vi "BasicTestWithIFw.vi"() -> ()   [LabVIEW 2015]
uses:
  SVPWM/SwitchPositions.ctl
  <vilib>/Platform/TimedLoop/XDataNode/timing_clust.ctl
  <vilib>/Platform/TimedLoop/XDataNode/nitl_modes.ctl
  <vilib>/Platform/TimedLoop/XDataNode/wakeup.ctl
  <vilib>/rvi/FXPMathLib/FxpSinAndCos/subVIs/nifxpmath_SinAndCos_SimConfig.ctl
  <vilib>/rvi/Emulation/niFpgaGetClockAttributes.vi
  <vilib>/rvi/Emulation/niFpgaSctlEmulationGetInTimedLoop.vi
  <vilib>/rvi/Emulation/niFpgaEmulationReportErrorSimple.vi
  <vilib>/rvi/FXPMathLib/FxpSinAndCos/simVIs/DllFxpSinAndCosTemp_sub.vi
  <vilib>/rvi/Emulation/niFpgaProcessEmulError.vi
  <vilib>/rvi/Emulation/niFpgaCriticalErrorInLSC.vi
  <vilib>/rvi/DataTransferAndStorage/Container/Common/niFpgaContainerExecOnDevCompGetState.vi
  <vilib>/rvi/Emulation/niFpgaEmulationIsFPGAContextNoSignature.vi
  <vilib>/rvi/DataTransferAndStorage/Container/Common/niFpgaContainerGetUniqueNameForEmu.vi
  <vilib>/rvi/Memory/Memory_Emulation/niFpgaMemoryEmulationCacheClearOnFirstRun.vi
  <vilib>/rvi/Memory/Memory_Emulation/nirvimemoryEmulationManagerCache_MakeExclusive.vi
  <vilib>/rvi/Memory/Memory_Emulation/niFpgaMemoryEmulationValidateCache.vi
  <vilib>/rvi/Memory/Memory_Emulation/nirvimemoryEmulationManagerCache_InsertValue.vi
  <vilib>/Utility/error.llb/Clear Errors.vi
  <vilib>/rvi/Memory/Memory_Emulation/nirvimemoryEmulationManagerCache_ReleaseExclusive.vi
  <vilib>/rvi/Memory/Memory_Emulation/nirvimemoryEmulationManagerCache_GetValue.vi
  <vilib>/rvi/Memory/Memory_Emulation/nirvimemoryEmulationManagerCache_SetValue.vi
  <vilib>/rvi/eio/common/nirviEmuTemplateMethod_errors.vi
  <vilib>/rvi/FXPMathLib/FxpSinAndCos/XNode/nifxpmath_SinAndCos.xnode
  <vilib>/Platform/TimedLoop/XDataNode/XDataNode.xnode
  <vilib>/rvi/DataTransferAndStorage/Container/XNode/niFpgaContainer.xnode
  <vilib>/rvi/DataTransferAndStorage/Register/Emulation/niFpgaRegisterEmulationRefIn.vi
  <vilib>/eio/EIONode/EIONode.xnode
  <vilib>/Platform/TimedLoop/XDataNode/XDNodeRunTimeDep.lvlib
  SVPWM/SVPWM.lvlib
  SVPWM/AddressSpace.lvclass
  <instrlib>/_niInstr/Instruction Framework/v1/FPGA/Top Level Bus/Register Configuration/Register Configuration.lvclass
  <instrlib>/_niInstr/FIFO Register Bus/v1/FPGA/niInstr FIFO Register Bus v1 FPGA.lvclass
panel:
  out "Period":u32
  out "Deadtime":u8
  in  "fifo reg bus ctrl 0":u32
  out "fifo reg bus status 0":u32
  out "fifo reg bus data 0":u64
  out "SwitchPositions":T1
  out "Sector":u8
  in  "enable":bool
  in  "engauge":bool
  in  "freq":sgl
  in  "modulation":fxp<+/-,16,2>=1.0
  out "As":sgl
  out "Bs":sgl
  out "Cs":sgl
  out "alpha":sgl
  out "beta":sgl
  in  "Count(Ticks)":u32=400
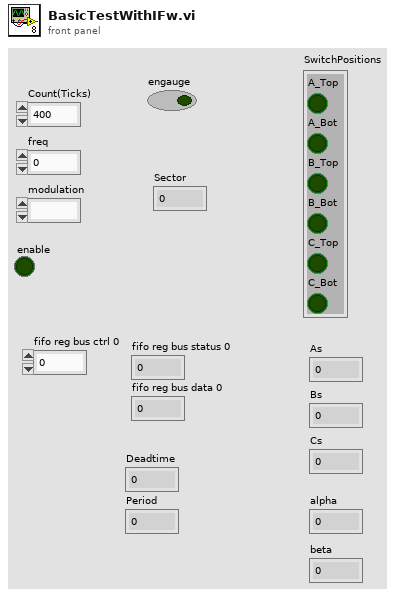
[diagram p1: front panel]
types:
  T1 = typedef "SVPWM.lvlib/SwitchPositions.ctl" = cluster{"A_Top":bool, "A_Bot":bool, "B_Top":bool, "B_Bot":bool, "C_Top":bool, "C_Bot":bool}
  T2 = typedef "XDNodeRunTimeDep.lvlib/timing_clust.ctl" = cluster{"Expected End [f-1]":u64, "Actual End [f-1]":u64, "Finished Late? [f-1]":bool, "Expected End [i-1]":u64, "Actual End [i-1]":u64, "Finished Late? [i-1]":bool, "Expected Start [i]":u64, "Actual Start [i]":u64, "Expected Start [f]":u64, "Actual Start [f]":u64, "Source Name":string, "Structure Name":string, "Period":i64, "Deadline":i64, "Offset":i64, "Start":i64, "Priority":i32, "Timeout":i32, "Mode":T3, "Wakeup Reason":T4, "Error":errorcluster, "Source Type":string, "Secondary Source Type":string, "Global End Time":u64, "Global Start Time":u64, "Frame Duration":u64, "Iteration Duration":u64, "Assigned CPU":i32, "I/O Scan Engine Mode":u32}
  T3 = typedef "XDNodeRunTimeDep.lvlib/nitl_modes.ctl" = enum32{"No Change", "Process missed periods, maintain original phase", "Discard missed periods, maintain original phase", "Process missed periods, ignore original phase", "Discard missed periods, ignore original phase"}
  T4 = typedef "XDNodeRunTimeDep.lvlib/wakeup.ctl" = enum32{"Normal", "Aborted", "Asynchronous wakeup", "Timing source error", "Timed loop error", "Timeout"}
  T5 = typedef "SVPWM.lvlib/Parameters.ctl" = cluster{"Deadtime":refnum<k21>, "Period":refnum<k21>}
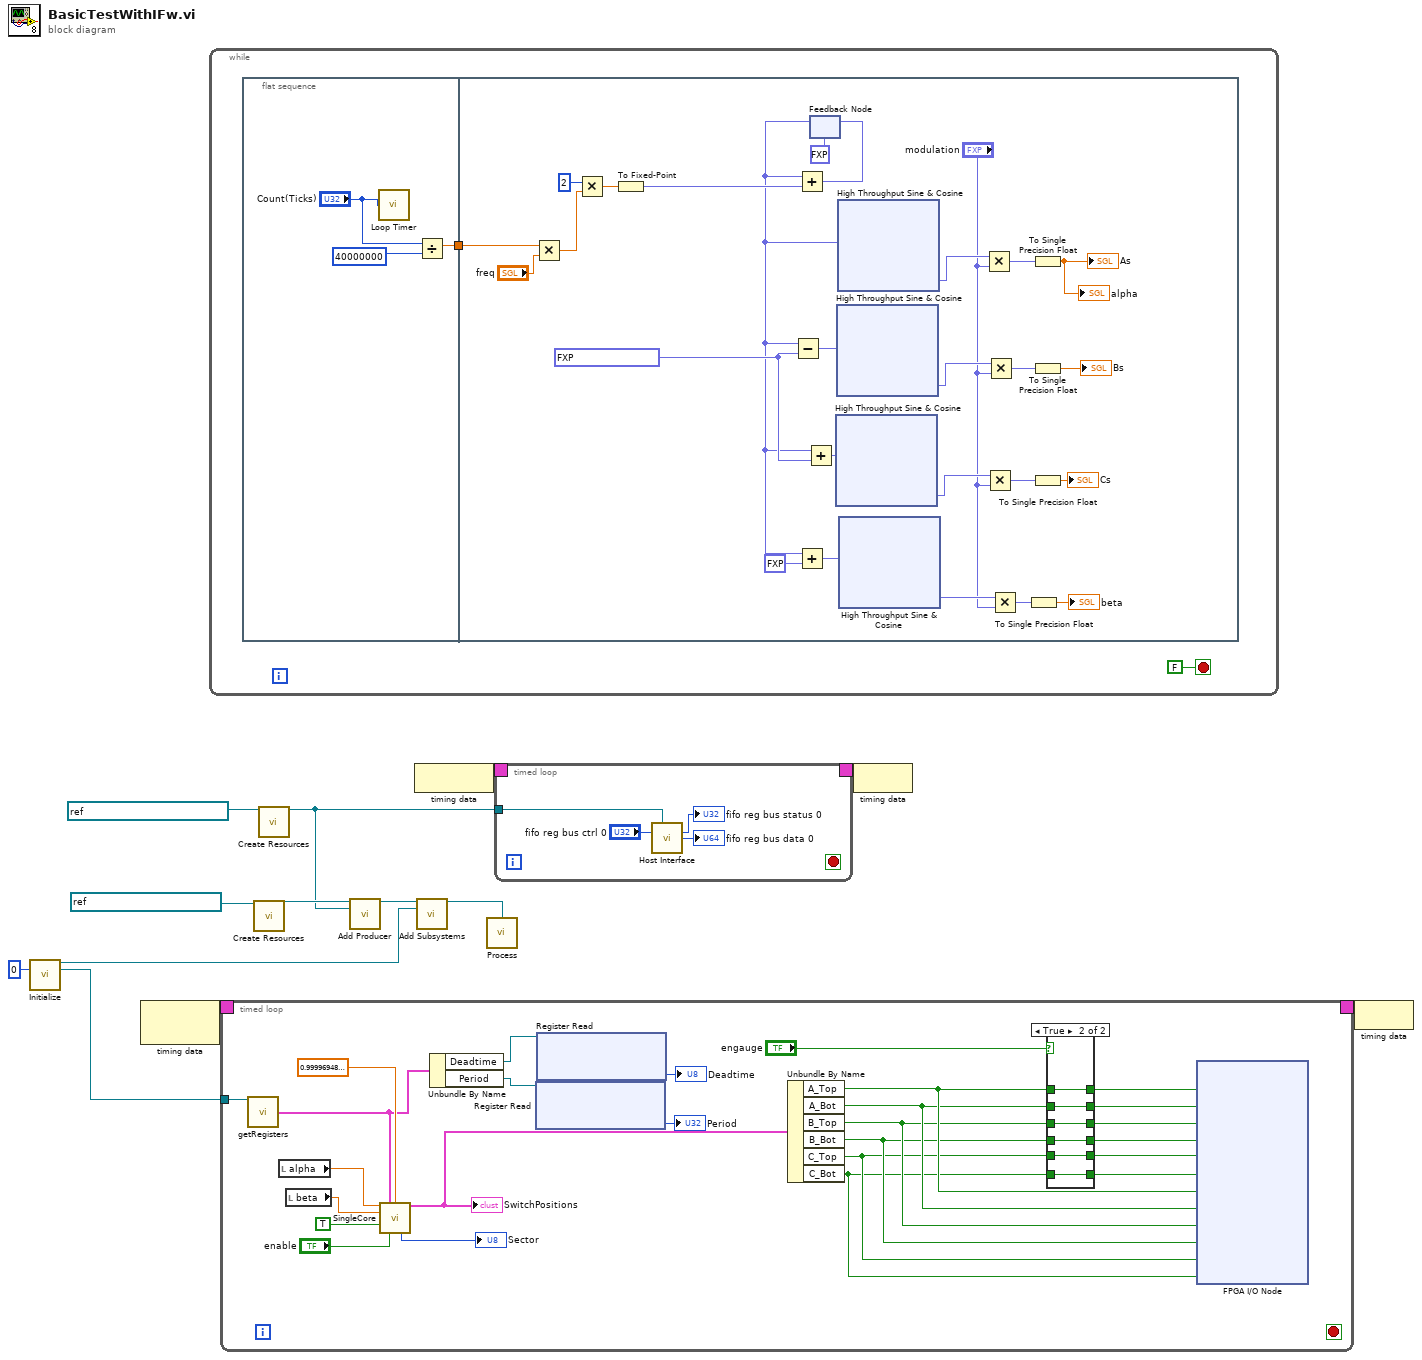
[diagram p0: block diagram]
diagram:
  n1 = call "Initialize.vi"("instance"=u8 0) -> ("subsystem"=w7:refnum<class "Single Address Space Collection.lvclass">, "AddressSpace"=w6:refnum<class "AddressSpace.lvclass">)  [unwired: 13 in]
  n2 = node-c288() -> (w13:T2)  [unwired: 1 in]
  n3 = while {
    stop <- FALSE stop-if-true
    n4 = flat-sequence {
      tunnel: [w16] -> w14
      tunnel: w14 -> [w37]
      frame #0 {
        n5 = call "Loop Timer"("Count(Ticks)"="Count(Ticks)") -> ()  [unwired: 1 out]
        n6 = Divide(x="Count(Ticks)", y=u32 40000000) -> (x/y=w16:sgl)
      }
      frame #1 {
        w44 = fxp<+/-,16,1> 0.666656494140625 ("x (pi)")
        n7 = Multiply(x=w37, y="freq") -> (x*y=w39:sgl)
        n8 = Multiply(x=i16 2, y=w39) -> (x*y=w30:sgl)
        n9 = To Fixed-Point(number=w30) -> (fixed-point=w29:fxp<+/-,32,16>)  [unwired: 1 in]
        n10 = feedback #1(fxp<+/-,16,1> 0.0 ("x (pi)")) -> (w24:fxp<+/-,16,1>)
        n11 = Subtract(x=w24, y=w44) -> (x-y=w43:fxp<+/-,17,2>)
        n12 = Add(x=w24, y=w29) -> (x+y=w40:fxp<+/-,16,1>)
        n13 = Add(x=w24, y=fxp<+/-,16,1> 0.5) -> (x+y=w25:fxp<+/-,17,2>)
        n14 = Add(x=w24, y=w44) -> (x+y=w45:fxp<+/-,17,2>)
        n15 = feedback-in #1(w40) -> ()
        n16 = xnode "High Throughput Sine & Cosine"("x (pi)"=w45) -> ("cos(x)"=w28:fxp<+/-,16,2>)  [unwired: 1 out]
        n17 = xnode "High Throughput Sine & Cosine"("x (pi)"=w43) -> ("cos(x)"=w27:fxp<+/-,16,2>)  [unwired: 1 out]
        n18 = xnode "High Throughput Sine & Cosine"("x (pi)"=w24) -> ("cos(x)"=w26:fxp<+/-,16,2>)  [unwired: 1 out]
        n19 = xnode "High Throughput Sine & Cosine"("x (pi)"=w25) -> ("cos(x)"=w21:fxp<+/-,16,2>)  [unwired: 1 out]
        n20 = Multiply(x=w26, y="modulation") -> (x*y=w36:fxp<+/-,32,4>)
        n21 = Multiply(x=w28, y="modulation") -> (x*y=w31:fxp<+/-,32,4>)
        n22 = Multiply(x=w27, y="modulation") -> (x*y=w33:fxp<+/-,32,4>)
        n23 = Multiply(x=w21, y="modulation") -> (x*y=w19:fxp<+/-,32,4>)
        n24 = To Single Precision Float(number=w19) -> (single precision float=→"beta":sgl)
        n25 = To Single Precision Float(number=w36) -> (single precision float=→"As" →"alpha":sgl)
        n26 = To Single Precision Float(number=w33) -> (single precision float=→"Bs":sgl)
        n27 = To Single Precision Float(number=w31) -> (single precision float=→"Cs":sgl)
      }
    }
  }
  n28 = timed-loop {
    timing: w13 -> [_]
    timing-out: [_] -> w12
    tunnel: w6 -> [w171]
    stop <- _ stop-if-true
    n29 = call "getRegisters.vi"("AddressSpace in"=w171) -> ("Parameters"=w170:T5)  [unwired: 13 in, 1 out]
    n30 = local read "alpha"() -> (w174:sgl)
    n31 = local read "beta"() -> (w173:sgl)
    n32 = call "SingleCore.vi"("alpha"=w174, "Parameters"=w170, "ref_max"=sgl 0.9999695, "beta"=w173, "input valid"=TRUE ("enable"), "enable"="enable") -> ("SwitchPositions"=w175:T1, "Sector"=→"Sector":u8)  [unwired: 7 in, 1 out]
    "SwitchPositions" <- w175
    n33 = Unbundle By Name(w170) -> ("Deadtime"=w169:refnum<k21>, "Period"=w168:refnum<k21>)
    n34 = xnode "Register Read"("Register In"=w168) -> ("Data"=→"Period":u32)  [unwired: 1 out]
    n35 = xnode "Register Read"("Register In"=w169) -> ("Data"=→"Deadtime":u8)  [unwired: 1 out]
    n36 = Unbundle By Name(w175) -> ("A_Top"=w187:bool, "A_Bot"=w185:bool, "B_Top"=w183:bool, "B_Bot"=w181:bool, "C_Top"=w179:bool, "C_Bot"=w177:bool)
    n37 = case shown="True" "engauge" {
      tunnel: w187 -> [_ w197]
      tunnel: [_ w197] -> w186
      tunnel: w185 -> [_ w196]
      tunnel: [_ w196] -> w184
      tunnel: w183 -> [_ w195]
      tunnel: [_ w195] -> w182
      tunnel: w181 -> [_ w194]
      tunnel: [_ w194] -> w180
      tunnel: w179 -> [_ w193]
      tunnel: [_ w193] -> w178
      tunnel: w177 -> [_ w192]
      tunnel: [_ w192] -> w176
      frame False {
      }
      frame True {
      }
    }
    n38 = xnode "FPGA I/O Node"("s2B / uTOPB"=w186, "s1B / uBOTB"=w184, "s4B / vTOPB"=w182, "s3B  / vBOTB"=w180, "s6B / wTOPB"=w178, "s5B / wBOTB"=w176, "uTOPB"=w187, "uBOTB"=w185, "vTOPB"=w183, "vBOTB"=w181, "wTOPB"=w179, "wBOTB"=w177) -> ()  [unwired: 12 in, 12 out]
  }
  n39 = call <instrlib>:"Create Resources.vi"("register clock"=refnum<k21> "40 MHz Onboard Clock") -> ("register configuration"=w11:refnum<class "Register Configuration.lvclass">)  [unwired: 14 in]
  n40 = call <instrlib>:"Create Resources.vi"("instruction fifo"=refnum<k21> "reg.host instruction fifo 0") -> ("fifo register bus"=w2:refnum<class "niInstr FIFO Register Bus v1 FPGA.lvclass">)  [unwired: 14 in]
  n41 = call <instrlib>:"Add Producer.vi"("register configuration in"=w11, "instruction producer"=w2) -> ("register configuration out"=w9:refnum<class "Register Configuration.lvclass">)  [unwired: 13 in]
  n42 = node-c288() -> (w5:T2)
  n43 = call <instrlib>:"Add Subsystems.vi"("register configuration in"=w9, "subsystems"=w7) -> ("register configuration out"=w8:refnum<class "Register Configuration.lvclass">)  [unwired: 13 in]
  n44 = call <instrlib>:"Process.vi"("register configuration"=w8) -> ()  [unwired: 15 in]
  n45 = timed-loop {
    timing: w5 -> [_]
    timing-out: [_] -> w4
    tunnel: w2 -> [w203]
    stop <- _ stop-if-true
    n46 = call <instrlib>:"Host Interface.vi"("fifo register bus"=w203, "fifo reg bus ctrl 0"="fifo reg bus ctrl 0") -> ("fifo reg bus status 0"=→"fifo reg bus status 0":u32, "fifo reg bus data 0"=→"fifo reg bus data 0":u64)  [unwired: 12 in]
  }
  n47 = node-c288(w4) -> ()
  n48 = node-c288(w12) -> ()
